vi "Calculate Flow Rate.vi"(11 "AirPump Controls":T1 {"Air Pump PWM" min=0 max=99.9 step=0.1 scale=0.0..100.0}) -> (3 "Flow Rate":i32)   [LabVIEW 2015]
uses:
  Controls/AirPump Controls.ctl
panel:
  out "output variable":i32
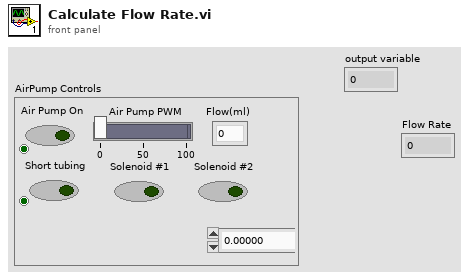
[diagram p1: front panel]
types:
  T1 = typedef "AirPump Controls.ctl" = cluster{"Air Pump PWM":sgl, "Solenoid #1":bool, "Solenoid #2":bool, "Air Pump On":bool, "Short tubing":bool, "Loflo Connected":bool, "Flow(ml)":u16, "Wait Active":bool}
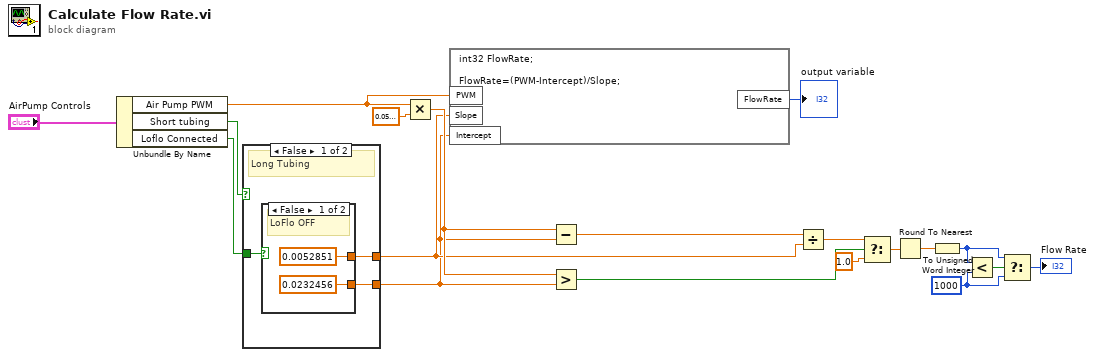
[diagram p0: block diagram]
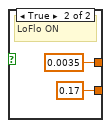
[diagram p2: hidden frame]
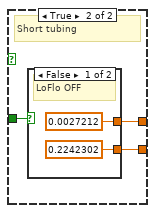
[diagram p3: hidden frame]
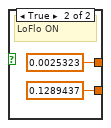
[diagram p4: hidden frame]
diagram:
  w18 = 1000 ("Numeric in")
  n1 = Unbundle By Name("AirPump Controls") -> ("Air Pump PWM"=w1:sgl, "Short tubing"=w6:bool, "Loflo Connected"=w7:bool)
  n2 = case shown="False" w6 {
    tunnel: w7 -> [w20 w27]
    tunnel: [w21 w29] -> w4
    tunnel: [w22 w28] -> w5
    frame False {
      # "Long Tubing"
      n3 = case shown="False" w20 {
        tunnel: [0.0232456 0.17] -> w21
        tunnel: [0.0052851 0.0035] -> w22
        frame False {
          # "LoFlo OFF"
        }
        frame True {
          # "LoFlo ON"
        }
      }
    }
    frame True {
      # "Short tubing"
      n4 = case shown="False" w27 {
        tunnel: [0.2242302 0.1289437] -> w29
        tunnel: [0.0027212 0.0025323] -> w28
        frame False {
          # "LoFlo OFF"
        }
        frame True {
          # "LoFlo ON"
        }
      }
    }
  }
  n5 = Multiply(x=w1, y=sgl 0.05) -> (x*y=w11:sgl)
  n6 = formula code="int32 FlowRate; \n\nFlowRate=(PWM-Intercept)/Slope;"("PWM"=w1, "Slope"=w5, "Intercept"=w4) -> ("FlowRate"=→"output variable":i32)
  n7 = Subtract(x=w11, y=w4) -> (x-y=w9:dbl)
  n8 = Greater?(x=w11, y=w4) -> (0:w12:bool)
  n9 = Divide(x=w9, y=w5) -> (x/y=w14:dbl)
  n10 = Select(t=w14, s=w12, f=1.0) -> (s? t:f=w13:dbl)
  n11 = Round To Nearest(number=w13) -> (nearest integer value=w10:dbl)
  n12 = To Unsigned Word Integer(number=w10) -> (unsigned 16bit integer=w17:u16)
  n13 = Less?(x=w17, y=w18) -> (x < y?=w16:bool)
  n14 = Select(t=w17, s=w16, f=w18) -> (s? t:f=→"Flow Rate":i32)
